vi "RunByReference.vi"(8 "error in (no error)":errorcluster, 10 "BW icon in":T1, 11 "Color icon in":T1) -> (0 "error out":errorcluster, 1 "Error code out":i32, 2 "BW icon out":T1, 3 "Color icon out":T1)   [LabVIEW 2021, in "IconEditorInterface.lvlib" / "IconEditorInterface.lvclass"]
uses:
  <resource>/plugins/NIIconEditor/UI/Interface class/IconEditorInterface.lvclass
  <vilib>/picture/picture.llb/imagedata.ctl
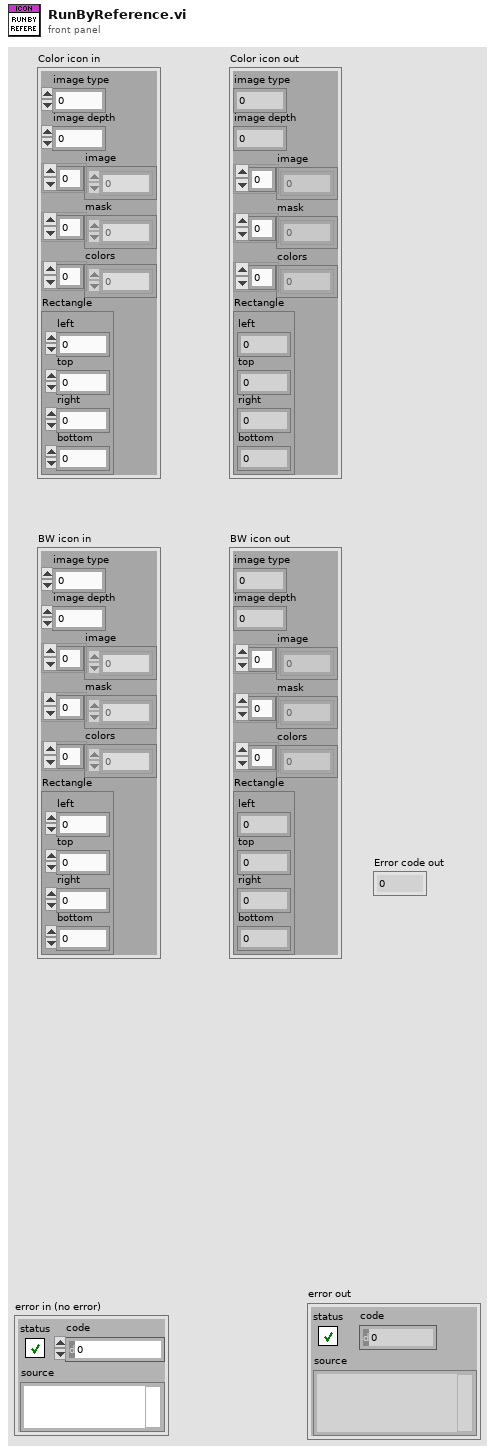
[diagram p1: front panel]
types:
  T1 = typedef "imagedata.ctl" = cluster{"image type":i32, "image depth":i32, "image":u8[], "mask":u8[], "colors":u32[], "Rectangle":cluster{"left":i16, "top":i16, "right":i16, "bottom":i16}}
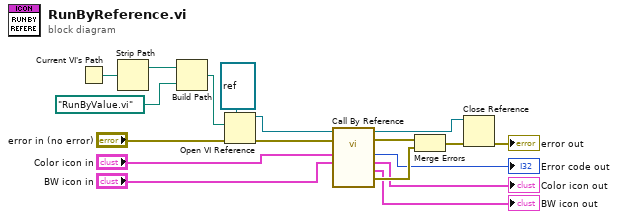
[diagram p0: block diagram]
diagram:
  n1 = Current VI's Path() -> (path=w6:path)
  n2 = Strip Path(path=w6) -> (stripped path=w5:path)  [unwired: 1 out]
  n3 = Build Path(base path=w5, name or relative path=path "RunByValue.vi") -> (appended path=w3:path)
  n4 = Open VI Reference(type specifier VI Refnum (for type only)=refnum<vi> refnum, vi path=w3, error in (no error)="error in (no error)") -> (vi reference=w7:refnum<vi>, error out=w1:errorcluster)  [unwired: 3 in]
  n5 = call-by-ref "?"(reference=w7, error in=w1, "BW icon in"="BW icon in", "Color icon in"="Color icon in") -> (reference out=w16:refnum<vi>, error out=w15:errorcluster, 0:"error out"=w13:errorcluster, "BW icon out"=→"BW icon out":T1, "Color icon out"=→"Color icon out":T1, "Error code out"=→"Error code out":i32)  [unwired: 6 in]
  n6 = Merge Errors(w15, w13) -> (w14:errorcluster)
  n7 = Close Reference(reference=w16, error in (no error)=w14) -> (error out=→"error out":errorcluster)
